vi "Initialize.vi"() -> (14 "Fatal Error Out":T11, 15 "State Out":T1)   [LabVIEW 2021, in "myRIO AudioOut N Samples Open.xnode"]
uses:
  <vilib>/myRIO/Instrument Drivers/Onboard IO/AudioOut Block/vis/myRIO AudioOut N Samples Open.xnode
  <vilib>/XNodeSupport/XNodeErrorCluster.ctl
  <vilib>/myRIO/Instrument Drivers/Onboard IO/AudioOut Block/vis/State.ctl
  <vilib>/myRIO/Common/Instrument Driver Framework/Utilities/typedefs/myRIOXPeripheral.ctl
  <vilib>/XNodeSupport/XNodeTerm4Array.ctl
  <vilib>/XNodeSupport/XNodeTerm4.ctl
  <vilib>/XNodeSupport/XNodeString.ctl
  <vilib>/XNodeSupport/XNodeVariant.ctl
  <vilib>/XNodeSupport/XNodeRect32.ctl
  <vilib>/XNodeSupport/XNodeInt.ctl
  <vilib>/XNodeSupport/XNodeBool.ctl
  <vilib>/XNodeSupport/XNodeTermDirection.ctl
  <vilib>/myRIO/Instrument Drivers/Onboard IO/AudioOut Block/typedefs/AudioOut Block Reference.ctl
  <vilib>/myRIO/Common/Instrument Driver Framework/Utilities/typedefs/myRIO Generic Hardware Reference.ctl
  <vilib>/myRIO/Common/Instrument Driver Framework/Utilities/typedefs/Hardware Version Enum.ctl
  <vilib>/myRIO/Common/Instrument Driver Framework/Utilities/typedefs/myRIO v1.0 Reference.ctl
  <vilib>/myRIO/Common/Instrument Driver Framework/Utilities/typedefs/Generic FPGA Reference.ctl
  <vilib>/myRIO/Common/Instrument Driver Framework/myRIO v1.0/AudioOut Block/typedefs/AudioOut Block Channels List.ctl
  <vilib>/myRIO/Common/Instrument Driver Framework/myRIO v1.0/AudioOut Block/typedefs/AudioOut Block Channels Enum.ctl
  <vilib>/myRIO/Common/Instrument Driver Framework/Utilities/typedefs/Analog Scaling Constants.ctl
  <vilib>/myRIO/Common/Instrument Driver Framework/Utilities/vis/myRIOXGlobal.vi
  <vilib>/XNodeSupport/NI_XNodeSupport.lvlib
  <vilib>/myRIO/Instrument Drivers/Onboard IO/AudioOut Block/AudioOut Block.lvlib
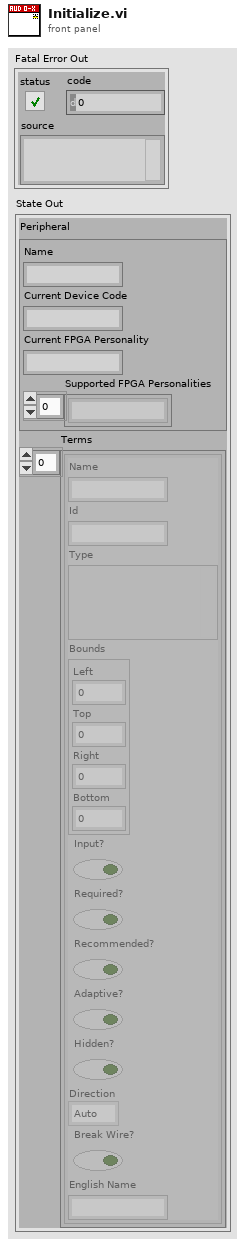
[diagram p1: front panel]
types:
  T1 = typedef "myRIO AudioOut N Samples Open.xnode/State.ctl" = cluster{"Peripheral":T2, "Terms":T3}
  T2 = typedef "myRIOXPeripheral.ctl" = cluster{"Name":string, "Current Device Code":string, "Current FPGA Personality":string, "Supported FPGA Personalities":string[]}
  T3 = typedef "NI_XNodeSupport.lvlib/XNodeTerm4Array.ctl" = T4[]
  T4 = typedef "NI_XNodeSupport.lvlib/XNodeTerm4.ctl" = cluster{"Name":T5, "Id":T5, "Type":T6, "Bounds":T7, "Input?":T9, "Required?":T9, "Recommended?":T9, "Adaptive?":T9, "Hidden?":T9, "Direction":T10, "Break Wire?":T9, "English Name":T5}
  T5 = typedef "NI_XNodeSupport.lvlib/XNodeString.ctl" = string
  T6 = typedef "NI_XNodeSupport.lvlib/XNodeVariant.ctl" = variant
  T7 = typedef "NI_XNodeSupport.lvlib/XNodeRect32.ctl" = cluster{"Left":T8, "Top":T8, "Right":T8, "Bottom":T8}
  T8 = typedef "NI_XNodeSupport.lvlib/XNodeInt.ctl" = i32
  T9 = typedef "NI_XNodeSupport.lvlib/XNodeBool.ctl" = bool
  T10 = typedef "NI_XNodeSupport.lvlib/XNodeTermDirection.ctl" = enum32{"Auto", "Up", "Down", "Left", "Right", "Center"}
  T11 = typedef "NI_XNodeSupport.lvlib/XNodeErrorCluster.ctl" = errorcluster
  T12 = typedef "AudioOut Block.lvlib/AudioOut Block Reference.ctl" = cluster{"myRIO Reference":T13, "AudioOut (N Samples) Channels List":T17, "AudioOut (N Samples) Scaling Constants List":T19[]}
  T13 = typedef "myRIO Generic Hardware Reference.ctl" = cluster{"myRIO Model":T14, "myRIO Hardware Reference":T15}
  T14 = typedef "Hardware Version Enum.ctl" = enum16{"Unknown", "myRIO-1900", "myRIO-1950", "roboRIO", "NI ELVIS RIO CM", "ELVIS III"}
  T15 = typedef "myRIO v1.0 Reference.ctl" = cluster{"Generic FPGA Reference":T16, "Allow multiple opens":bool}
  T16 = typedef "Generic FPGA Reference.ctl" = refnum<k20>
  T17 = typedef "AudioOut Block Channels List.ctl" = T18[]
  T18 = typedef "AudioOut Block Channels Enum.ctl" = enum16{"Not Connected", "AudioOut/Left (N Samples)", "AudioOut/Right (N Samples)"}
  T19 = typedef "Analog Scaling Constants.ctl" = cluster{"LSB Weight (Volts)":dbl, "Offset (Volts)":dbl, "Signed?":bool}
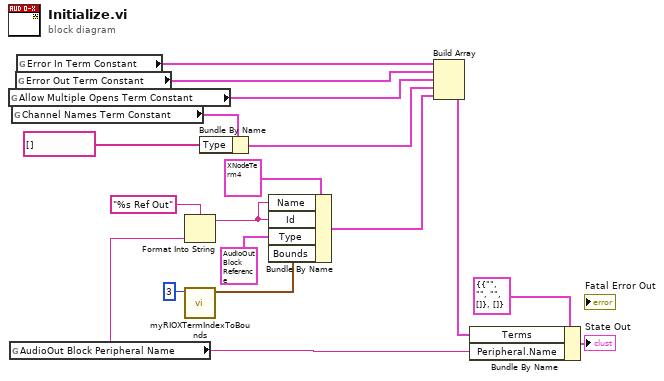
[diagram p0: block diagram]
diagram:
  n1 = global read "myRIOXGlobal.vi" "Allow Multiple Opens Term Constant"() -> (w13:T4)
  n2 = global read "myRIOXGlobal.vi" "AudioOut Block Peripheral Name"() -> (w3:string)
  n3 = global read "myRIOXGlobal.vi" "Channel Names Term Constant"() -> (w7:T4)
  n4 = global read "myRIOXGlobal.vi" "Error Out Term Constant"() -> (w14:T4)
  n5 = global read "myRIOXGlobal.vi" "Error In Term Constant"() -> (w15:T4)
  n6 = Format Into String(format string="%s Ref Out" ("Name"), w3) -> (resulting string=w11:string)  [unwired: 2 in, 1 out]
  n7 = call <vilib>:"myRIOXTermIndexToBounds.vi"("Index"=3) -> ("Bounds"=w10:T7)  [unwired: 10 in]
  n8 = Bundle By Name(cluster=w7, "Type"=tag[] [] ("myRIO AudioOut Block Channel List")) -> (w5:T4)
  n9 = Bundle By Name(cluster=T4 {"Name"="", "Id"="", "Type"=variant, "Bounds"={"Left"=0, "Top"=0, "Right"=0, "Bottom"=0}, "Input?"=FALSE, "Required?"=FALSE, "Recommended?"=TRUE, "Adaptive?"=FALSE, "Hidden?"=FALSE, "Direction"=enum."Auto", "Break Wire?"=FALSE, "English Name"=""} ("Channel Names Term Constant"), "Name"=w11, "Id"=w11, "Type"=T12 {"myRIO Reference"={"myRIO Model"=enum."Unknown", "myRIO Hardware Reference"={"Generic FPGA Reference"=refnum, "Allow multiple opens"=FALSE}}, "AudioOut (N Samples) Channels List"=[], "AudioOut (N Samples) Scaling Constants List"=[]} ("AudioOut Block Reference"), "Bounds"=w10) -> (w4:T4)
  n10 = Build Array(w15, w14, w13, w5, w4) -> (w2:T4[])
  n11 = Bundle By Name(cluster=T1 {"Peripheral"={"Name"="", "Current Device Code"="", "Current FPGA Personality"="", "Supported FPGA Personalities"=[]}, "Terms"=[]} ("State Out"), "Terms"=w2, "Peripheral.Name"=w3) -> (→"State Out":T1)
